vi "Volts to FXP Codes.vi"(0 "scaling coefficients":T1[](array[typedef]), 5 "channel index":u8, 7 "level (V)":dbl, 9 "Range (V)":dbl, 11 "Center (V)":dbl) -> (4 "level (fxp)":fxp<+/-,18,1> format="%.18g", 6 "range (fxp)":fxp<+/-,18,1> format="%.18g", 8 "Center (fxp)":fxp<+/-,18,1> format="%.18g")   [LabVIEW 2021, in "Device Session.lvclass"]
uses:
  Device Session.lvclass
  <instrlib>/_niInstr/Multirecord Acquisition/Interface/v1/Host/Public/Scaling Coefficient.ctl
  <instrlib>/_niInstr/Multirecord Acquisition/Interface/v1/Host/niInstr Multirecord Acquisition v1 Host.lvclass
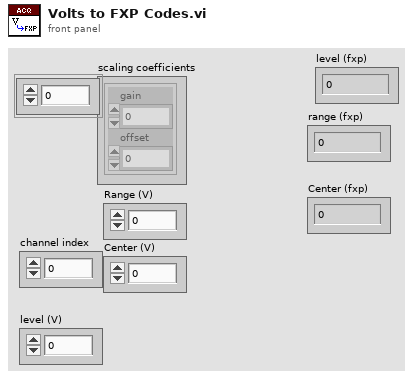
[diagram p1: front panel]
types:
  T1 = typedef "niInstr Multirecord Acquisition v1 Host.lvclass/Scaling Coefficient.ctl" = cluster{"gain":dbl, "offset":dbl}
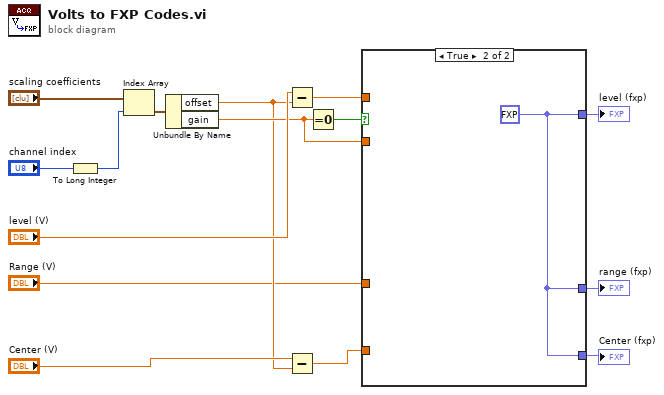
[diagram p0: block diagram]
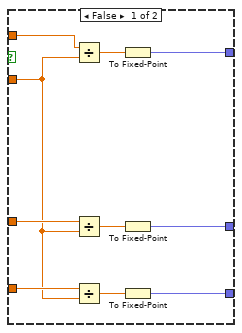
[diagram p2: hidden frame]
diagram:
  n1 = To Long Integer(number="channel index") -> (32bit integer=w7:i32)
  n2 = Index Array(array="scaling coefficients", index=w7) -> (element=w13:T1)
  n3 = Unbundle By Name(w13) -> ("offset"=w4:dbl, "gain"=w10:dbl)
  n4 = Subtract(x="level (V)", y=w4) -> (x-y=w14:dbl)
  n5 = Subtract(x="Center (V)", y=w4) -> (x-y=w5:dbl)
  n6 = Equal To 0?(x=w10) -> (x = 0?=w12:bool)
  n7 = case shown="True" w12 {
    tunnel: w14 -> [w25 _]
    tunnel: [w23 w26] -> w11
    tunnel: w10 -> [w18 _]
    tunnel: w5 -> [w22 _]
    tunnel: [w20 w26] -> w3
    tunnel: "Range (V)" -> [w19 _]
    tunnel: [w16 w26] -> w1
    frame False {
      n8 = Divide(x=w25, y=w18) -> (x/y=w24:dbl)
      n9 = Divide(x=w19, y=w18) -> (x/y=w17:dbl)
      n10 = Divide(x=w22, y=w18) -> (x/y=w21:dbl)
      n11 = To Fixed-Point(number=w24) -> (fixed-point=w23:fxp<+/-,18,1>)  [unwired: 1 in]
      n12 = To Fixed-Point(number=w17) -> (fixed-point=w16:fxp<+/-,18,1>)  [unwired: 1 in]
      n13 = To Fixed-Point(number=w21) -> (fixed-point=w20:fxp<+/-,18,1>)  [unwired: 1 in]
    }
    frame True {
      w26 = fxp<+/-,18,1> 0.0
    }
  }
  "level (fxp)" <- w11
  "Center (fxp)" <- w3
  "range (fxp)" <- w1
